vi "wfm_feature update_active_plot.vi"(8 "error in (no error)":errorcluster, 10 "index of element":i32, 11 "wfm_feature in":refnum<class "wfm_feature.lvclass">) -> (0 "error out":errorcluster, 3 "wfm_feature out":refnum<class "wfm_feature.lvclass">)   [LabVIEW 2018, in "wfm_feature.lvclass"]
uses:
  wfm_feature.lvclass
  wfm_feature.lvclass/wfm_feature.ctl
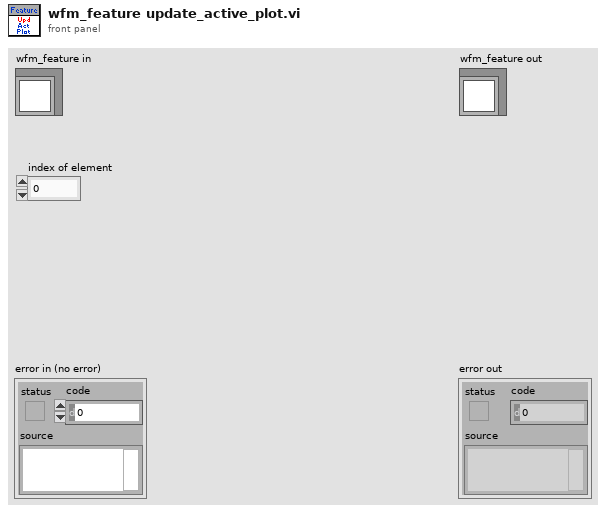
[diagram p1: front panel]
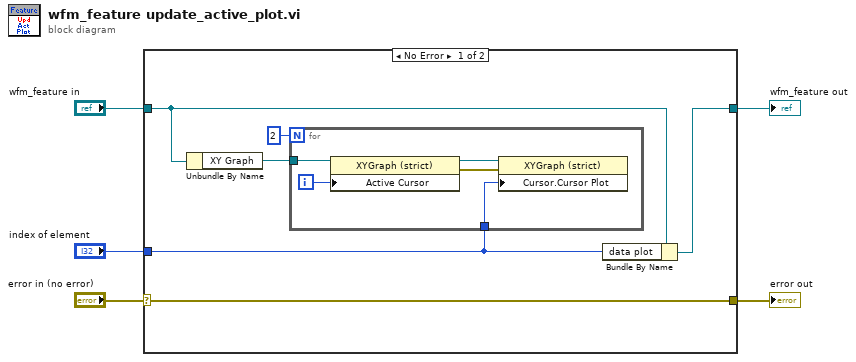
[diagram p0: block diagram]
diagram:
  n1 = case shown="No Error" "error in (no error)" {
    selector: "error in (no error)" -> [w11 w18]
    tunnel: [w11 w18] -> w4
    tunnel: [w7 w17] -> w2
    tunnel: "wfm_feature in" -> [w8 w17]
    tunnel: "index of element" -> [w6 _]
    frame No Error {
      n2 = Unbundle By Name(w8) -> ("XY Graph"=w10:refnum<vi>)
      n3 = for {
        N: 2 -> [_]
        tunnel: w10 -> [w16]
        tunnel: w6 -> [w13]
        i -> [w12]
        n4 = property class="XYGraph (strict)"(reference=w16, "Active Cursor"=w12) -> (reference out=w15:refnum<vi>, error out=w14:errorcluster)  [unwired: 1 in]
        n5 = property class="XYGraph (strict)"(reference=w15, error in=w14, "Cursor.Cursor Plot"=w13) -> ()  [unwired: 2 out]
      }
      n6 = Bundle By Name(cluster=w8, "data plot"=w6) -> (w7:refnum<class "wfm_feature.lvclass">)
    }
    frame Error {
    }
  }
  "error out" <- w4
  "wfm_feature out" <- w2
